vi "2L18_nc_vers_z_bi.vi"(3 "Niveau de confiance (1- alpha)":dbl=0.95 format="%.2f") -> (0 "-z (alpha/2)":dbl format="%.2f", 1 "z (apha/2)":dbl format="%.2f")   [LabVIEW 2010, in "lv_02.lvlib"]
doc: "Pour un niveau de confiance NC= 1-alpha, on calcule la variable réduite z en répartissant alpha de manière bilatérale."
uses:
  lv_02.lvlib
  1A-z-invdist.vi
panel:
  # "Risque alpha bilatéral"
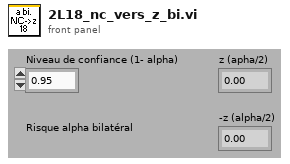
[diagram p1: front panel]
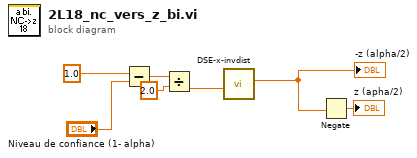
[diagram p0: block diagram]
diagram:
  n1 = Subtract(x=1.0, y="Niveau de confiance (1- alpha)") -> (x-y=w4:dbl)
  n2 = Divide(x=w4, y=2.0) -> (x/y=w2:dbl)
  n3 = call-poly "DSE-x-invdist.vi"("F(z)"=w2) -> ("z"=w1:dbl)  [unwired: 8 in, 2 out]
  "-z (alpha/2)" <- w1
  n4 = Negate(x=w1) -> (-x=→"z (apha/2)":dbl)
